vi "DialogUsingEvents 1.vi"() -> (2 "Attachment path":path, 3 "Cancelled?":bool)   [LabVIEW 2015]
doc: "Use this template to create a dialog box with event handling."
panel:
  in  "Attachment path":path
  in  "Cancel":bool
  in  "OK":bool
  # "Choose the path for attachment saving\npress cancel for default path\nPress cancel in case of the master device"
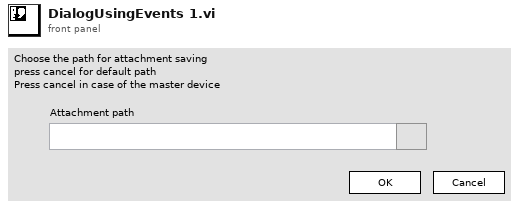
[diagram p1: front panel]
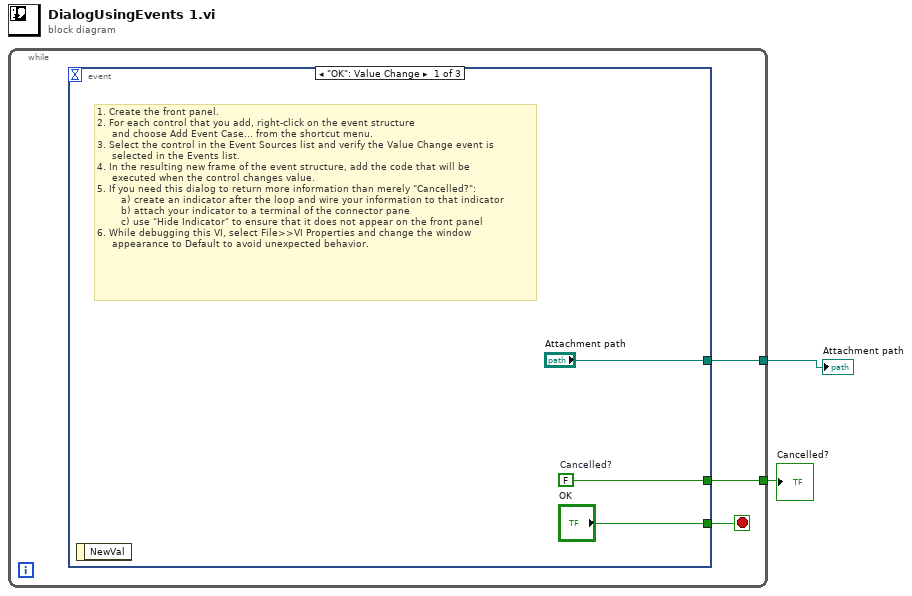
[diagram p0: block diagram]
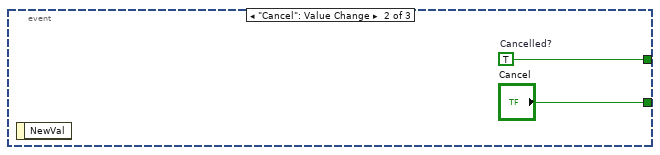
[diagram p2: hidden frame]
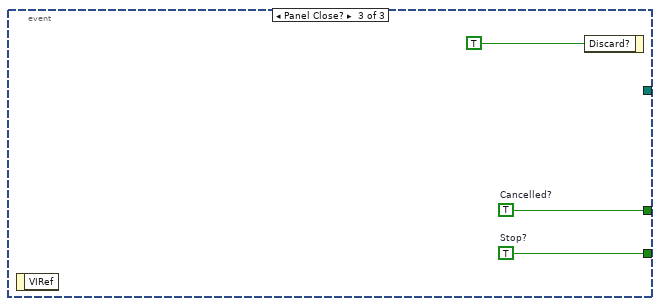
[diagram p3: hidden frame]
diagram:
  n1 = while {
    tunnel: [w4] -> w2
    tunnel: [w3] -> w1
    stop <- w5 stop-if-true
    n2 = event shown="[0] \"OK\": Value Change" {
      selector: _ -> [_ _ _]
      dyn-events: _ -> [_ _ _]
      timeout: _ -> [_ _ _]
      tunnel: ["OK" "Cancel" w12] -> w5
      tunnel: [w8 w10 w11] -> w4
      tunnel: ["Attachment path" _ _] -> w3
      event "OK": Value Change {
        w8 = FALSE  # Cancelled?
        # "1. Create the front panel.\n2. For each control that you add, right-click on the event structure \n     and choose Add Event Case... from the shortcut menu.\n3. Select the control in the Event Sources list and verify the Value Change event is \n     selected in the Events list.\n4. In the resulting new frame of the event structure, add the code that will be \n     executed when the control changes value.\n5. If you need this dialog to return more information than merely \"Cancelled?\":\n        a) create an indicator after the loop and wire your information to that indicator\n        b) attach your indicator to a terminal of the connector pane\n        c) use \"Hide Indicator\" to ensure that it does not appear on the front panel\n6. While debugging this VI, select File>>VI Properties and change the window \n     appearance to Default to avoid unexpected behavior."
        n3 = event-data() -> ()  [unwired: 1 in, 1 out]
      }
      event "Cancel": Value Change {
        w10 = TRUE  # Cancelled?
        n4 = event-data() -> ()  [unwired: 1 in, 1 out]
      }
      event Panel Close? {
        w11 = TRUE  # Cancelled?
        w12 = TRUE  # Stop?
        n5 = event-data() -> ()  [unwired: 1 in, 1 out]
        n6 = event-data("Discard?"=TRUE) -> ()  [unwired: 1 in, 1 out]
      }
    }
  }
  "Cancelled?" <- w2
  "Attachment path" <- w1
